vi "detDirWall.vi"(1 "Radius":i32, 2 "Y-cord":i32, 3 "X-cord":i32, 4 "Source Image":T1(plugin-control)) -> (0 "Angle dir":i32)   [LabVIEW 2009, in "ImageAnalysis.lvlib"]
uses:
  ImageAnalysis.lvlib
  <vilib>/vision/NI_Vision_Development_Module.lvlib
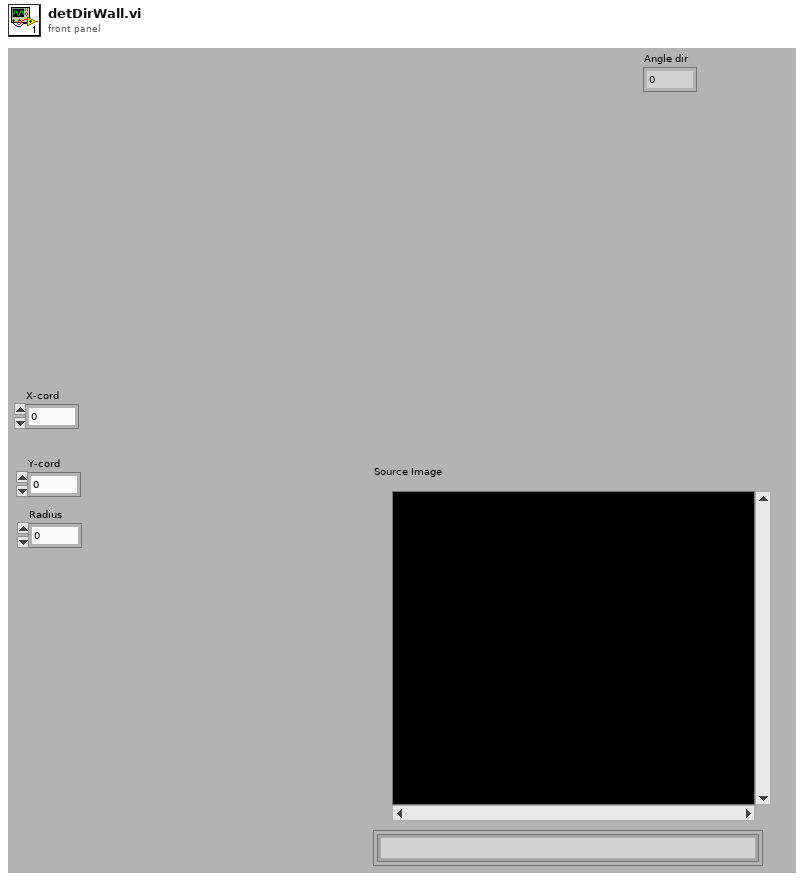
[diagram p1: front panel]
types:
  T1 = typedef "IMAQ Image.ctl" = refnum<image>
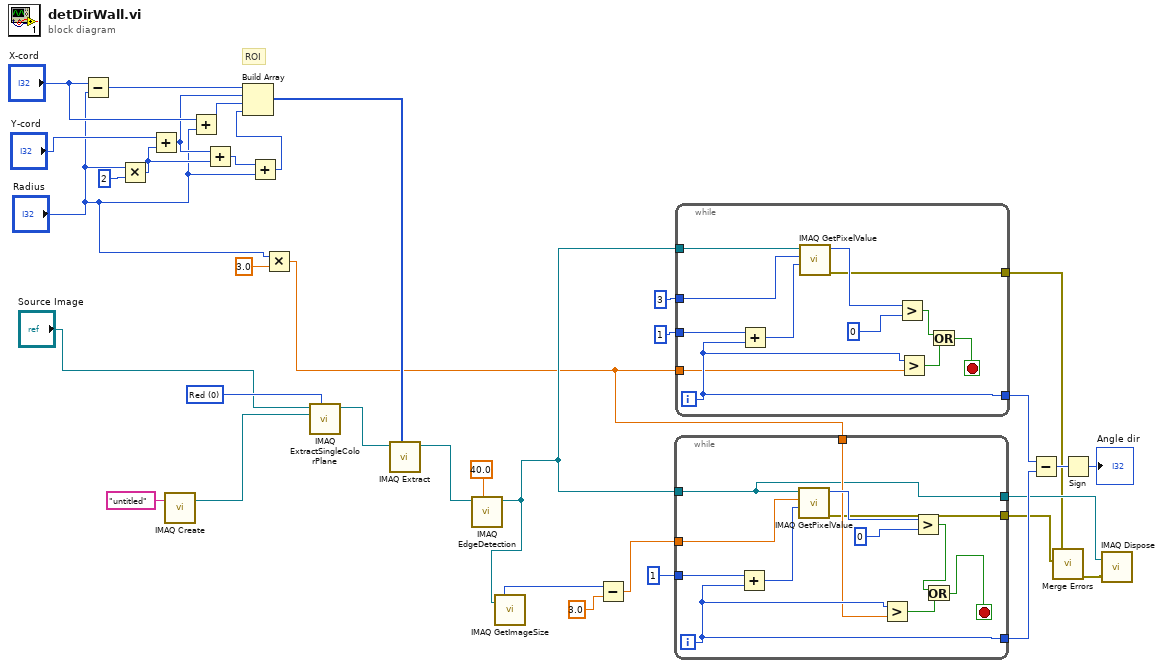
[diagram p0: block diagram]
diagram:
  w35 = 0 items=["Red", "Green", "Blue", "Hue", "Saturation", "Luminance", "Value", "Intensity"] ("Color Plane")
  # "ROI"
  n1 = Subtract(x="X-cord", y="Radius") -> (x-y=w22:i32)
  n2 = Multiply(x="Radius", y=2) -> (x*y=w16:i32)
  n3 = Add(x="Y-cord", y=w16) -> (x+y=w17:i32)
  n4 = call "IMAQ Create"("Image Name"="untitled") -> ("New Image"=w12:T1)  [unwired: 4 in, 1 out]
  n5 = Add(x="X-cord", y="Radius") -> (x+y=w21:i32)
  n6 = Add(x=w17, y=w16) -> (x+y=w15:i32)
  n7 = Add(x=w15, y="Radius") -> (x+y=w14:i32)
  n8 = Build Array(w22, w17, w21, w14) -> (w10:i32[])
  n9 = Multiply(x="Radius", y=3.0) -> (x*y=w5:dbl)
  n10 = call "IMAQ ExtractSingleColorPlane"("Color Plane"=w35, "Image Dst"=w12, "Image Src"="Source Image") -> ("Image Dst Out"=w8:T1)  [unwired: 7 in, 1 out]
  n11 = call "IMAQ Extract"("Optional Rectangle"=w10, "Image Src"=w8) -> ("Image Dst Out"=w9:T1)  [unwired: 8 in, 1 out]
  n12 = call "IMAQ EdgeDetection"("Threshold Value"=sgl 40.0, "Image Src"=w9) -> ("Image Dst Out"=w26:T1)  [unwired: 8 in, 1 out]
  n13 = call "IMAQ GetImageSize"("Image"=w26) -> ("X Resolution"=w24:i32)  [unwired: 3 in, 2 out]
  n14 = Subtract(x=w24, y=3.0) -> (x-y=w23:dbl)
  n15 = while {
    tunnel: w26 -> [w37]
    tunnel: [w39] -> w29
    tunnel: w23 -> [w45]
    tunnel: 1 ("Y Coordinate") -> [w44]
    tunnel: w5 -> [w38]
    tunnel: [w37] -> w4
    tunnel: [w36] -> w2
    i -> [w39]
    stop <- w40 stop-if-true
    n16 = Add(x=w44, y=w39) -> (x+y=w43:i32)
    n17 = call "IMAQ GetPixelValue"("Image"=w37, "X Coordinate"=w45, "Y Coordinate"=w43) -> ("Pixel Value (U8)"=w47:u8, "error out"=w36:errorcluster)  [unwired: 3 in, 3 out]
    n18 = Greater?(x=w39, y=w38) -> (0:w42:bool)
    n19 = Greater?(x=w47, y=u8 0) -> (0:w41:bool)
    n20 = Or(x=w41, y=w42) -> (x .or. y?=w40:bool)
  }
  n21 = while {
    tunnel: w26 -> [w49]
    tunnel: [w51] -> w30
    tunnel: 3 ("X Coordinate") -> [w57]
    tunnel: 1 ("Y Coordinate") -> [w56]
    tunnel: w5 -> [w50]
    tunnel: [w48] -> w3
    i -> [w51]
    stop <- w52 stop-if-true
    n22 = Add(x=w56, y=w51) -> (x+y=w55:i32)
    n23 = call "IMAQ GetPixelValue"("Image"=w49, "X Coordinate"=w57, "Y Coordinate"=w55) -> ("Pixel Value (U8)"=w59:u8, "error out"=w48:errorcluster)  [unwired: 3 in, 3 out]
    n24 = Greater?(x=w59, y=u8 0) -> (0:w53:bool)
    n25 = Greater?(x=w51, y=w50) -> (0:w54:bool)
    n26 = Or(x=w53, y=w54) -> (x .or. y?=w52:bool)
  }
  n27 = Subtract(x=w30, y=w29) -> (x-y=w27:i32)
  n28 = call <vilib>:"Merge Errors.vi"("error in 2 (no error)"=w2, "error in 1 (no error)"=w3) -> ("error out"=w1:errorcluster)  [unwired: 5 in]
  n29 = Sign(1:w27) -> (0:→"Angle dir":i32)
  n30 = call "IMAQ Dispose"("Image"=w4, "error in (no error)"=w1) -> ()  [unwired: 4 in, 1 out]
